vi "Load.vi"(8 "error in (no error)":errorcluster, 11 "Project File":path) -> (0 "error out":errorcluster, 3 "Project":refnum<class "Project.lvclass">)   [LabVIEW 2015, in "Project.lvclass"]
uses:
  Project.lvclass
  <vilib>/xml/Load XML String.vi
  <vilib>/xml/Close Reference(Node).vi
  <vilib>/xml/NI_XML.lvlib
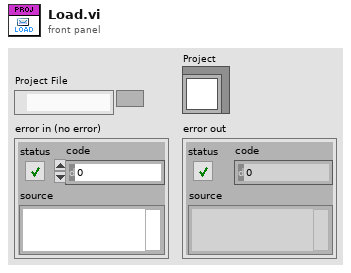
[diagram p1: front panel]
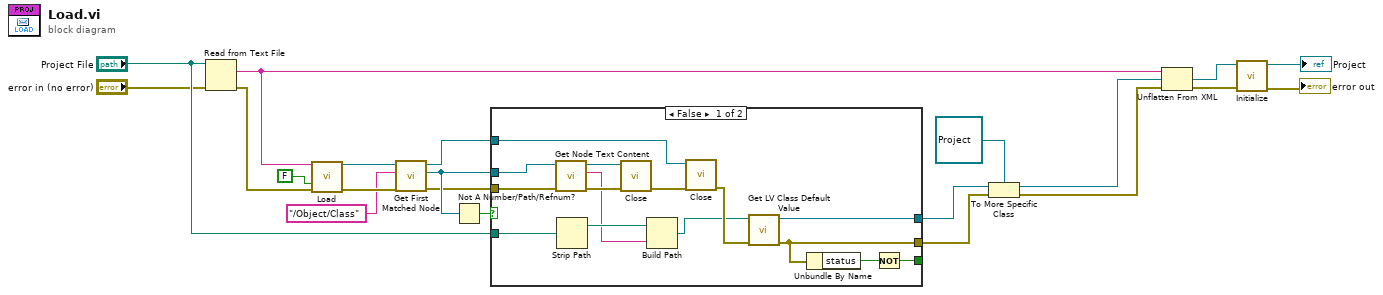
[diagram p0: block diagram]
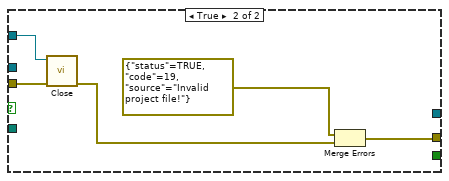
[diagram p2: hidden frame]
diagram:
  n1 = Read from Text File(file (use dialog)="Project File", error in="error in (no error)") -> (text=w21:string, error out=w12:errorcluster)  [unwired: 2 in, 2 out]
  n2 = call-poly <vilib>:"Load.vi"("XML string"=w21, "load external DTD (True)"=FALSE, "error in (no error)"=w12) -> ("DOM document out"=w19:refnum<k20>, "error out"=w18:errorcluster)  [unwired: 10 in, 1 out]
  n3 = call <vilib>:"Get First Matched Node.vi"("error in (no error)"=w18, "XPath expression"="/Object/Class", "node in"=w19) -> ("error out"=w14:errorcluster, "node result"=w15:refnum<k20>, "node out"=w13:refnum<k20>)  [unwired: 6 in]
  n4 = Not A Number/Path/Refnum?(number/path/refnum=w15) -> (NaN/Path/Refnum?=w16:bool)
  n5 = case shown="False" w16 {
    tunnel: w15 -> [w36 _]
    tunnel: w14 -> [w35 w41]
    tunnel: w13 -> [w31 w40]
    tunnel: "Project File" -> [w30 _]
    tunnel: [w27 w37] -> w11
    tunnel: [w22 _] -> w10
    tunnel: [w26 _] -> _
    frame False {
      n6 = call <vilib>:"Get Node Text Content.vi"("error in (no error)"=w35, "node in"=w36) -> ("error out"=w33:errorcluster, "node text"=w24:string, "node out"=w34:refnum<k20>)  [unwired: 7 in]
      n7 = Strip Path(path=w30) -> (stripped path=w29:path)  [unwired: 1 out]
      n8 = call-poly <vilib>:"Close.vi"("error in (no error)"=w33, "node"=w34) -> ("error out"=w32:errorcluster)  [unwired: 7 in]
      n9 = Build Path(base path=w29, name or relative path=w24) -> (appended path=w23:path)
      n10 = call-poly <vilib>:"Close.vi"("error in (no error)"=w32, "node"=w31) -> ("error out"=w28:errorcluster)  [unwired: 7 in]
      n11 = call <vilib>:"Get LV Class Default Value.vi"("error in (no error)"=w28, "class path"=w23) -> ("error out"=w27:errorcluster, "object"=w22:refnum<class>)  [unwired: 8 in]
      n12 = Unbundle By Name(w27) -> ("status"=w25:bool)
      n13 = Not(x=w25) -> (.not. x?=w26:bool)
    }
    frame True {
      n14 = call-poly <vilib>:"Close.vi"("error in (no error)"=w41, "node"=w40) -> ("error out"=w38:errorcluster)  [unwired: 7 in]
      n15 = Merge Errors(errorcluster {"status"=TRUE, "code"=19, "source"="Invalid project file!"} ("error out"), w38) -> (w37:errorcluster)
    }
  }
  n16 = To More Specific Class(target class=refnum<class "Project.lvclass"> refnum ("Project.lvclass"), reference=w10, error in=w11) -> (specific class reference=w6:refnum<class "Project.lvclass">, error out=w5:errorcluster)
  n17 = Unflatten From XML(xml string=w21, type=w6, error in (no error)=w5) -> (value=w3:refnum<class "Project.lvclass">, error out=w4:errorcluster)
  n18 = call-dynamic "Initialize.vi"("error in (no error)"=w4, "ProjectBase in"=w3) -> ("error out"=→"error out":errorcluster, "ProjectBase out"=→"Project":refnum<class "Project.lvclass">)  [unwired: 8 in]
